vi "Grab and Basic Attributes.vi"() -> ()   [LabVIEW 2011]
doc: "The Grab and Basic Attributes example VI allows the user to view the current attributes and settings, update attribute settings, acquire images continuously, and display the images in an image control."
uses:
  <vilib>/vision/driver/NI_Vision_Acquisition_Software.lvlib
  <vilib>/vision/driver/IMAQdx.llb/IMAQdx Attribute Visibility.ctl
  resource/objmgr/imaqdx.rc
panel:
  in  "Set Attribute":bool
  in  "Attribute Value":string
  in  "Attribute Name":u32(ring) items=["CameraAttributes::AnalogControls::GainAuto", "CameraAttributes::AnalogControls::GainSelector", "CameraAttributes::AnalogControls::GainRaw", "CameraAttributes::AnalogControls::BlackLevelSelector", "CameraAttributes::AnalogControls::BlackLevelRaw", "CameraAttributes::AnalogControls::BalanceWhiteAuto", "CameraAttributes::AnalogControls::BalanceRatioSelector", "CameraAttributes::AnalogControls::BalanceRatioAbs", "CameraAttributes::AnalogControls::BalanceRatioRaw", "CameraAttributes::AnalogControls::GammaEnable", "CameraAttributes::AnalogControls::GammaSelector", "CameraAttributes::AnalogControls::Gamma", "CameraAttributes::AnalogControls::DigitalShift", "CameraAttributes::ImageFormat::PixelFormat", "CameraAttributes::ImageFormat::PixelSize", "CameraAttributes::ImageFormat::PixelColorFilter", "CameraAttributes::ImageFormat::PixelDynamicRangeMin", "CameraAttributes::ImageFormat::PixelDynamicRangeMax", "CameraAttributes::ImageFormat::ReverseX", "CameraAttributes::ImageFormat::TestImageSelector", "CameraAttributes::AOI::Width", "CameraAttributes::AOI::Height", "CameraAttributes::AOI::OffsetX", "CameraAttributes::AOI::OffsetY", "CameraAttributes::AOI::CenterX", "CameraAttributes::AOI::CenterY", "CameraAttributes::AcquisitionTrigger::AcquisitionMode", "CameraAttributes::AcquisitionTrigger::AcquisitionFrameCount", "CameraAttributes::AcquisitionTrigger::TriggerSelector", "CameraAttributes::AcquisitionTrigger::TriggerMode", "CameraAttributes::AcquisitionTrigger::TriggerSoftware", "CameraAttributes::AcquisitionTrigger::TriggerSource", "CameraAttributes::AcquisitionTrigger::TriggerActivation", "CameraAttributes::AcquisitionTrigger::ExposureMode", "CameraAttributes::AcquisitionTrigger::ExposureAuto", "CameraAttributes::AcquisitionTrigger::ExposureTimeAbs", "CameraAttributes::AcquisitionTrigger::ExposureTimeRaw", "CameraAttributes::AcquisitionTrigger::AcquisitionFrameRateEnable", "CameraAttributes::AcquisitionTrigger::AcquisitionFrameRateAbs", "CameraAttributes::AcquisitionTrigger::ResultingFrameRateAbs", "CameraAttributes::DigitalIO::LineSelector", "CameraAttributes::DigitalIO::LineMode", "CameraAttributes::DigitalIO::LineSource", "CameraAttributes::DigitalIO::LineInverter", "CameraAttributes::DigitalIO::LineDebouncerTimeAbs", "CameraAttributes::DigitalIO::LineStatus", "CameraAttributes::DigitalIO::LineStatusAll", "CameraAttributes::DigitalIO::UserOutputSelector", "CameraAttributes::DigitalIO::UserOutputValue", "CameraAttributes::DigitalIO::UserOutputValueAll", "CameraAttributes::TimerControls::TimerDelayTimebaseAbs", "CameraAttributes::TimerControls::TimerDurationTimebaseAbs", "CameraAttributes::TimerControls::TimerSelector", "CameraAttributes::TimerControls::TimerDelayAbs", "CameraAttributes::TimerControls::TimerDelayRaw", "CameraAttributes::TimerControls::TimerDurationAbs", "CameraAttributes::TimerControls::TimerDurationRaw", "CameraAttributes::TimerControls::TimerTriggerSource", "CameraAttributes::TimerControls::TimerTriggerActivation", "CameraAttributes::LUTControls::LUTSelector", "CameraAttributes::LUTControls::LUTEnable", "CameraAttributes::LUTControls::LUTIndex", "CameraAttributes::LUTControls::LUTValue", "CameraAttributes::DeviceInformation::DeviceVendorName", "CameraAttributes::DeviceInformation::DeviceModelName", "CameraAttributes::DeviceInformation::DeviceManufacturerInfo", "CameraAttributes::DeviceInformation::DeviceVersion", "CameraAttributes::DeviceInformation::DeviceFirmwareVersion", "CameraAttributes::DeviceInformation::DeviceID", "CameraAttributes::DeviceInformation::DeviceUserID", "CameraAttributes::DeviceInformation::SensorWidth", "CameraAttributes::DeviceInformation::SensorHeight", "CameraAttributes::DeviceInformation::WidthMax", "CameraAttributes::DeviceInformation::HeightMax", "CameraAttributes::ChunkDataStreams::ChunkModeActive", "CameraAttributes::ChunkDataStreams::ChunkSelector", "CameraAttributes::ChunkDataStreams::ChunkEnable", "CameraAttributes::ChunkData::ChunkStride", "CameraAttributes::ChunkData::ChunkOffsetX", "CameraAttributes::ChunkData::ChunkOffsetY", "CameraAttributes::ChunkData::ChunkWidth", "CameraAttributes::ChunkData::ChunkHeight", "CameraAttributes::ChunkData::ChunkDynamicRangeMin", "CameraAttributes::ChunkData::ChunkDynamicRangeMax", "CameraAttributes::ChunkData::ChunkPixelFormat", "CameraAttributes::ChunkData::ChunkTimestamp", "CameraAttributes::ChunkData::ChunkFramecounter", "CameraAttributes::ChunkData::ChunkLineStatusAll", "CameraAttributes::ChunkData::ChunkTriggerinputcounter", "CameraAttributes::ChunkData::ChunkLineTriggerIgnoredCounter", "CameraAttributes::ChunkData::ChunkFrameTriggerIgnoredCounter", "CameraAttributes::ChunkData::ChunkFrameTriggerCounter", "CameraAttributes::ChunkData::ChunkFramesPerTriggerCounter", "CameraAttributes::ChunkData::ChunkLineTriggerEndToEndCounter", "CameraAttributes::ChunkData::ChunkInputStatusAtLineTriggerBitsPerLine", "CameraAttributes::ChunkData::ChunkInputStatusAtLineTriggerIndex", "CameraAttributes::ChunkData::ChunkInputStatusAtLineTriggerValue", "CameraAttributes::ChunkData::ChunkShaftEncoderCounter", "CameraAttributes::ChunkData::ChunkPayloadCRC16", "CameraAttributes::EventsGeneration::EventSelector", "CameraAttributes::EventsGeneration::EventNotification", "CameraAttributes::EventsGeneration::ExposureEndEventData::ExposureEndEventStreamChannelIndex", "CameraAttributes::EventsGeneration::ExposureEndEventData::ExposureEndEventFrameID", "CameraAttributes::EventsGeneration::ExposureEndEventData::ExposureEndEventTimestamp", "CameraAttributes::EventsGeneration::LineStartOvertriggerEventData::LineStartOvertriggerEventStreamChannelIndex", "CameraAttributes::EventsGeneration::LineStartOvertriggerEventData::LineStartOvertriggerEventTimestamp", "CameraAttributes::EventsGeneration::FrameStartOvertriggerEventData::FrameStartOvertriggerEventStreamChannelIndex", "CameraAttributes::EventsGeneration::FrameStartOvertriggerEventData::FrameStartOvertriggerEventTimestamp", "CameraAttributes::EventsGeneration::AcquisitionStartOvertriggerEventData::AcquisitionStartOvertriggerEventStreamChannelIndex", "CameraAttributes::EventsGeneration::AcquisitionStartOvertriggerEventData::AcquisitionStartOvertriggerEventTimestamp", "CameraAttributes::EventsGeneration::FrameTimeoutEventData::FrameTimeoutEventStreamChannelIndex", "CameraAttributes::EventsGeneration::FrameTimeoutEventData::FrameTimeoutEventTimestamp", "CameraAttributes::EventsGeneration::EventOverrunEventData::EventOverrunEventStreamChannelIndex", "CameraAttributes::EventsGeneration::EventOverrunEventData::EventOverrunEventFrameID", "CameraAttributes::EventsGeneration::EventOverrunEventData::EventOverrunEventTimestamp", "CameraAttributes::UserSets::UserSetSelector", "CameraAttributes::UserSets::UserSetLoad", "CameraAttributes::UserSets::UserSetSave", "CameraAttributes::UserSets::DefaultSetSelector", "CameraAttributes::TransportLayer::PayloadSize", "CameraAttributes::AutoFunctions::AutoTargetValue", "CameraAttributes::AutoFunctions::AutoGainRawLowerLimit", "CameraAttributes::AutoFunctions::AutoGainRawUpperLimit", "CameraAttributes::AutoFunctions::AutoExposureTimeAbsLowerLimit", "CameraAttributes::AutoFunctions::AutoExposureTimeAbsUpperLimit", "CameraAttributes::AutoFunctions::AutoFunctionProfile", "CameraAttributes::AutoFunctions::AutoFunctionAOIs::AutoFunctionAOISelector", "CameraAttributes::AutoFunctions::AutoFunctionAOIs::AutoFunctionAOIWidth", "CameraAttributes::AutoFunctions::AutoFunctionAOIs::AutoFunctionAOIHeight", "CameraAttributes::AutoFunctions::AutoFunctionAOIs::AutoFunctionAOIOffsetX", "CameraAttributes::AutoFunctions::AutoFunctionAOIs::AutoFunctionAOIOffsetY"]
  in  "Camera Name":refnum<k21> caption="IMAQdx Session"
  out "Buffer Number":u32
  out "Image":T1(plugin-control)
  out "Frame Rate":dbl(knob) scale=0.0..100.0
  in  "Stop":bool
  # "Overview: Demonstrates how to view the current attributes and settings, update attribute settings, acquire images continuously, and display the images in an image control.\nRequirements: Vision Acquisition Software\nInstructions: \n1. Select the Camera Name\n2. Run the VI"
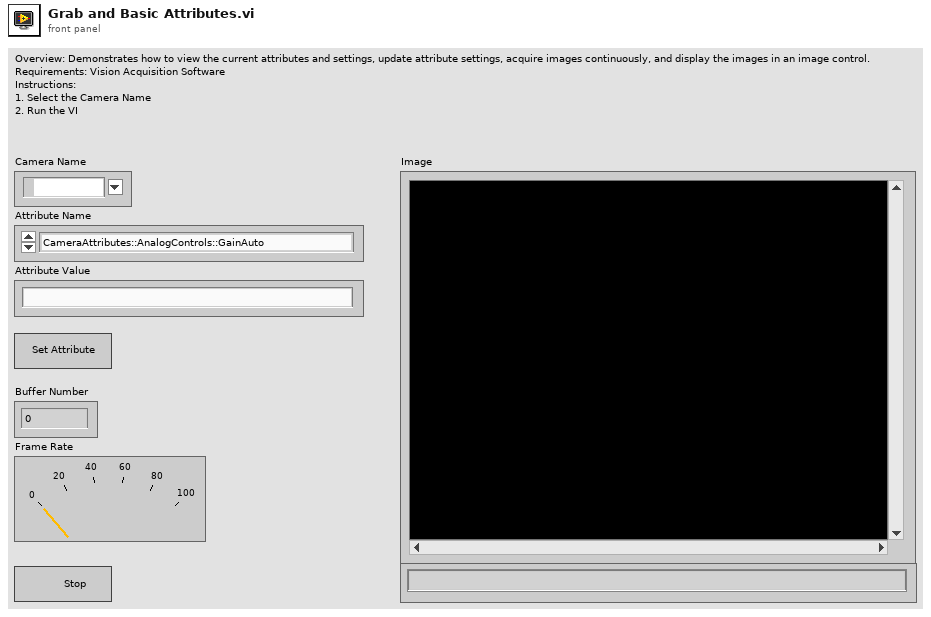
[diagram p1: front panel]
types:
  T1 = typedef "IMAQ Image.ctl" = refnum<image>
  T2 = typedef "NI_Vision_Acquisition_Software.lvlib/IMAQdx Attribute Visibility.ctl" = enum32{"Simple", "Intermediate", "Advanced"}
  T3 = typedef "IMAQdx.ctl" = refnum<k21>
  T4 = typedef "NI_Vision_Acquisition_Software.lvlib/IMAQdx Attribute Type.ctl" = enum32{"U32", "I64", "DBL", "String", "Enum", "Bool", "Command"}
  T5 = cluster{"Attribute Type":T4, "Readable":bool, "Writable":bool, "Attribute Name":string}[]
  T6 = enum8{"Enabled", "Disabled", "Disabled and Grayed Out"}
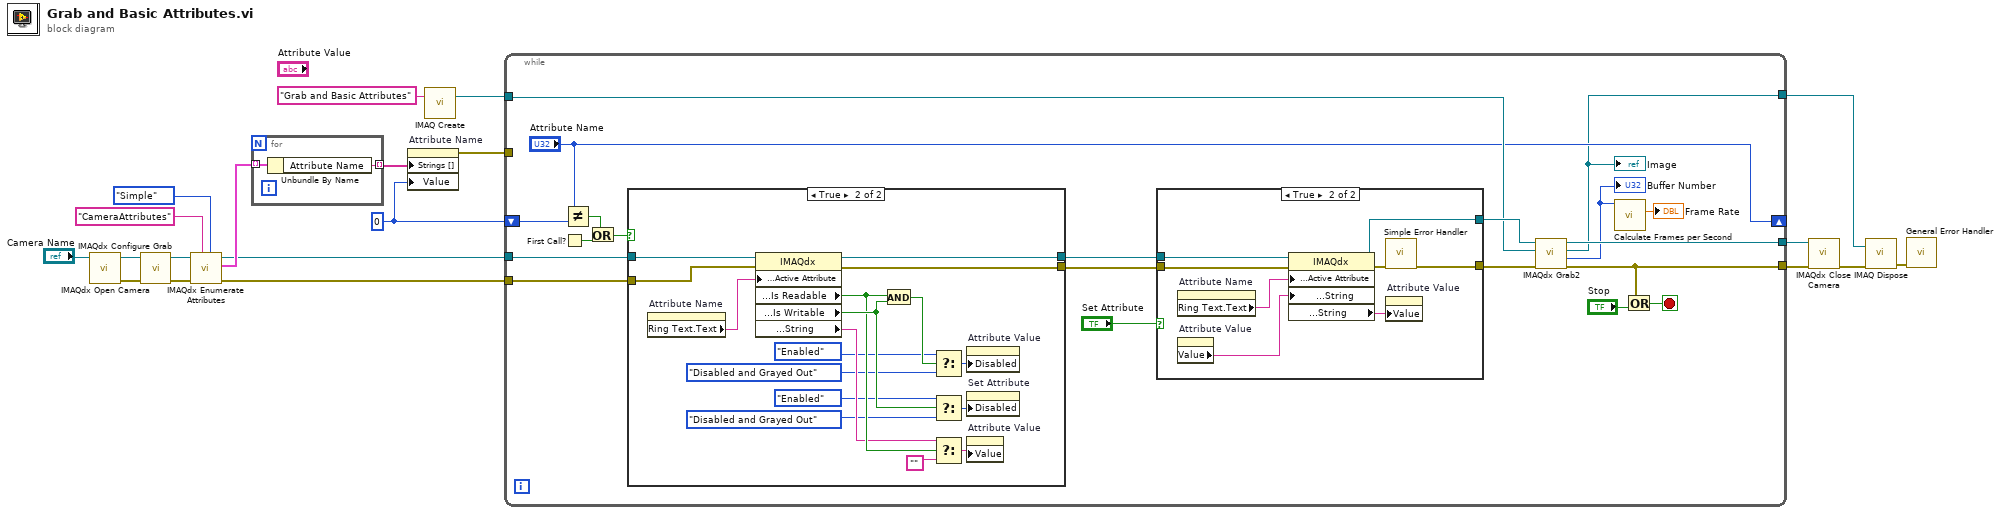
[diagram p0: block diagram]
diagram:
  w5 = u32 0 ("BufferInterval")
  n1 = call <vilib>:"IMAQdx Open Camera.vi"("Session In"="Camera Name") -> ("error out"=w20:errorcluster, "Session Out"=w19:T3)  [unwired: 2 in, 7 out]
  n2 = call <vilib>:"IMAQdx Configure Grab.vi"("error in"=w20, "Session In"=w19) -> ("error out"=w16:errorcluster, "Session Out"=w17:T3)  [unwired: 8 out]
  n3 = call <vilib>:"IMAQdx Enumerate Attributes.vi"("Visibility"=IMAQdx_Attribute_Visibility."Simple", "Root"="CameraAttributes", "error in"=w16, "Session In"=w17) -> ("error out"=w8:errorcluster, "Attribute Information Array"=w13:T5, "Session Out"=w9:T3)  [unwired: 5 out]
  n4 = for {
    tunnel: w13 -> [w22] mode=indexing
    tunnel: [w21] -> w12 mode=indexing
    n5 = Unbundle By Name(w22) -> ("Attribute Name"=w21:string)
  }
  n6 = property on="Attribute Name" class="Ring (strict)"("Strings []"=w12, "Value"=w5) -> (error out=w11:errorcluster)  [unwired: 2 in, 1 out]
  n7 = call "IMAQ Create"("Image Name"="Grab and Basic Attributes") -> ("New Image"=w10:T1)  [unwired: 3 in, 2 out]
  n8 = while {
    tunnel: w11 -> [_]
    tunnel: w9 -> [w37]
    tunnel: w10 -> [w34]
    tunnel: w8 -> [w24]
    shift-right: ["Attribute Name"] -> _
    shift-left: w5 -> [w40]
    tunnel: [w39] -> w7
    tunnel: [w38] -> w6
    tunnel: [w23] -> w1
    stop <- w42 stop-if-true
    n9 = First Call?() -> (First Call?: T/F=w31:bool)
    n10 = Not Equal?(x="Attribute Name", y=w40) -> (x != y?=w33:bool)
    n11 = Or(x=w33, y=w31) -> (x .or. y?=w32:bool)
    n12 = case shown="True" w32 {
      tunnel: w37 -> [w54 w62]
      tunnel: w24 -> [w53 w61]
      tunnel: [w54 w56] -> w26
      tunnel: [w53 w55] -> w25
      frame False {
      }
      frame True {
        n13 = property on="Attribute Name" class="Ring (strict)"() -> ("Ring Text.Text"=w67:string)  [unwired: 2 in, 2 out]
        n14 = property class="IMAQdx"(reference=w62, error in=w61, "Camera Attributes:Active Attribute"=w67) -> (reference out=w56:T3, error out=w55:errorcluster, "Camera Attributes:Is Readable"=w66:bool, "Camera Attributes:Is Writable"=w71:bool, "Camera Attributes:Value:String"=w65:string)
        n15 = And(x=w66, y=w71) -> (x .and. y?=w69:bool)
        n16 = Select(t=T6."Enabled" ("Disabled"), s=w69, f=T6."Disabled and Grayed Out" ("Disabled")) -> (s? t:f=w68:T6)
        n17 = Select(t=T6."Enabled" ("Disabled"), s=w71, f=T6."Disabled and Grayed Out" ("Disabled")) -> (s? t:f=w70:T6)
        n18 = Select(t=w65, s=w66, f="") -> (s? t:f=w64:string)
        n19 = property on="Attribute Value" class="Str"("Disabled"=w68) -> ()  [unwired: 2 in, 2 out]
        n20 = property on="Set Attribute" class="Bool"("Disabled"=w70) -> ()  [unwired: 2 in, 2 out]
        n21 = property on="Attribute Value" class="Str"("Value"=w64) -> ()  [unwired: 2 in, 2 out]
      }
    }
    n22 = case shown="True" "Set Attribute" {
      tunnel: w26 -> [w44 w48]
      tunnel: [w44 w47] -> w35
      tunnel: [w43 w46] -> w36
      tunnel: w25 -> [w43 w45]
      frame False {
      }
      frame True {
        n23 = property on="Attribute Name" class="Ring (strict)"() -> ("Ring Text.Text"=w49:string)  [unwired: 2 in, 2 out]
        n24 = property on="Attribute Value" class="Str"() -> ("Value"=w50:string)  [unwired: 2 in, 2 out]
        n25 = property class="IMAQdx"(reference=w48, error in=w45, "Camera Attributes:Active Attribute"=w49, "Camera Attributes:Value:String"=w50) -> (reference out=w47:T3, error out=w52:errorcluster, "Camera Attributes:Value:String"=w51:string)
        n26 = call <vilib>:"Simple Error Handler.vi"("error in (no error)"=w52) -> ("error out"=w46:errorcluster)  [unwired: 1 in, 7 out]
        n27 = property on="Attribute Value" class="Str"("Value"=w51) -> ()  [unwired: 2 in, 2 out]
      }
    }
    n28 = call <vilib>:"IMAQdx Grab2.vi"("error in"=w36, "Image In"=w34, "Session In"=w35) -> ("error out"=w38:errorcluster, "Buffer Number Out"=w28:u32, "Image Out"=w23:T1, "Session Out"=w39:T3)  [unwired: 5 in]
    "Image" <- w23
    "Buffer Number" <- w28
    n29 = call <vilib>:"Calculate Frames per Second.vi"("Buffer Number"=w28) -> ("Processed Frames/s"=→"Frame Rate":dbl)  [unwired: 8 in, 2 out]
    n30 = Or(x=w38, y="Stop") -> (x .or. y?=w42:bool)
  }
  n31 = call <vilib>:"IMAQdx Close Camera.vi"("error in"=w6, "Session In"=w7) -> ("error out"=w3:errorcluster)  [unwired: 9 out]
  n32 = call "IMAQ Dispose"("Image"=w1, "error in (no error)"=w3) -> ("error out"=w2:errorcluster)  [unwired: 4 in]
  n33 = call <vilib>:"General Error Handler.vi"("error in (no error)"=w2) -> ()  [unwired: 1 in, 14 out]
